vi "Graph Event Handler.vi"(11 "Graph Manager out 2":refnum<class "Graph Manager.lvclass">) -> (3 "Graph Manager out":refnum<class "Graph Manager.lvclass">)   [LabVIEW 2013, in "Graph Manager.lvclass"]
uses:
  Graph Manager.lvclass
  Graph Manager.lvclass/Graph Manager.ctl
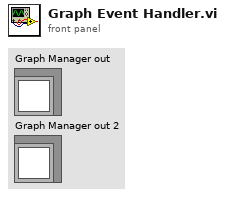
[diagram p1: front panel]
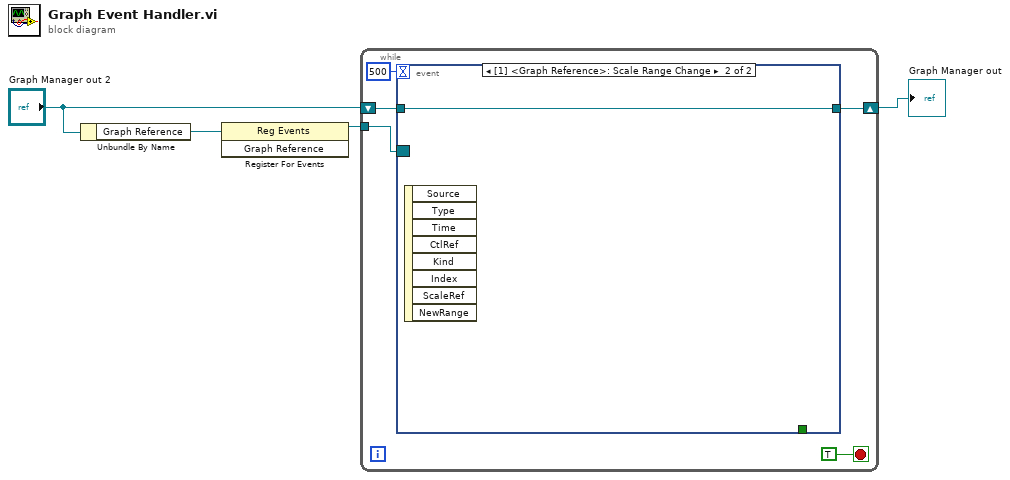
[diagram p0: block diagram]
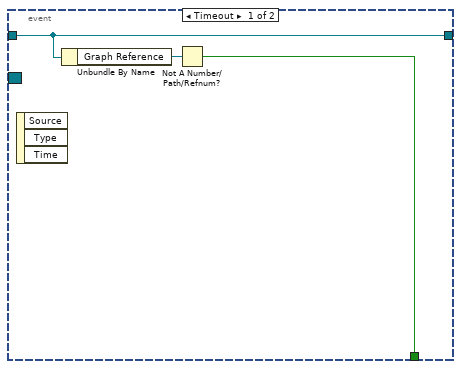
[diagram p2: hidden frame]
diagram:
  n1 = Unbundle By Name("Graph Manager out 2") -> ("Graph Reference"=w2:refnum<vi>)
  n2 = register-events(w2) -> (reference out=w1:refnum<event-registration>)  [unwired: 2 in, 1 out]
  n3 = while {
    shift-right: [w9] -> w4
    shift-left: "Graph Manager out 2" -> [w8]
    tunnel: w1 -> [w7]
    stop <- TRUE stop-if-true
    n4 = event shown="[1] <Graph Reference>: Scale Range Change" {
      selector: w7 -> [_ _]
      dyn-events: _ -> [_ _]
      timeout: 500 -> [_ _]
      tunnel: [w12 w13] -> w9
      tunnel: w8 -> [w12 w13]
      tunnel: [w10 _] -> _
      event Timeout {
        n5 = event-data() -> ()  [unwired: 1 in, 3 out]
        n6 = Unbundle By Name(w12) -> ("Graph Reference"=w11:refnum<vi>)
        n7 = Not A Number/Path/Refnum?(number/path/refnum=w11) -> (NaN/Path/Refnum?=w10:bool)
      }
      event Scale Range Change {
        n8 = event-data() -> ()  [unwired: 1 in, 8 out]
      }
    }
  }
  "Graph Manager out" <- w4
